vi "Construct Network Log Endpoint.vi"(8 "Max Number of Connections (-1)":i32=-1, 9 "Port":u16=7705, 10 "Net Address":u32, 11 "Logger to Write To":refnum<class "LoggerReference.lvclass">) -> (0 "error out":errorcluster, 3 "Network Sink Endpoint out":refnum<class "Network Sink Endpoint.lvclass">)   [LabVIEW 2017, in "Network Sink.lvlib" / "Network Sink Endpoint.lvclass"]
uses:
  <vilib>/gpm_packages/@cs/event-logger/Source/Network Sink/Network Sink Endpoint/Network Sink Endpoint.lvclass
  <vilib>/gpm_packages/@cs/event-logger/Source/Composed Log/LoggerReference/LoggerReference.lvclass
  <vilib>/gpm_packages/@cs/event-logger/Source/Network Sink/Network Sink Endpoint/Network Sink Endpoint.lvclass/Network Sink Endpoint.ctl
panel:
  # "The sink endpoint will stop itself with the logger shutdown - this output is only needed if you want to explicitly close the endpoint."
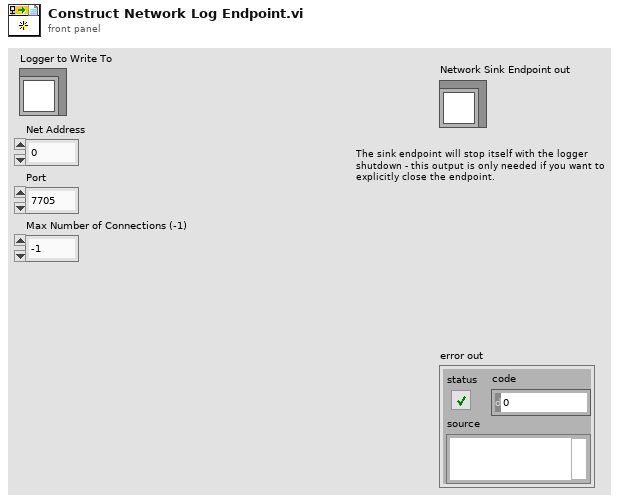
[diagram p1: front panel]
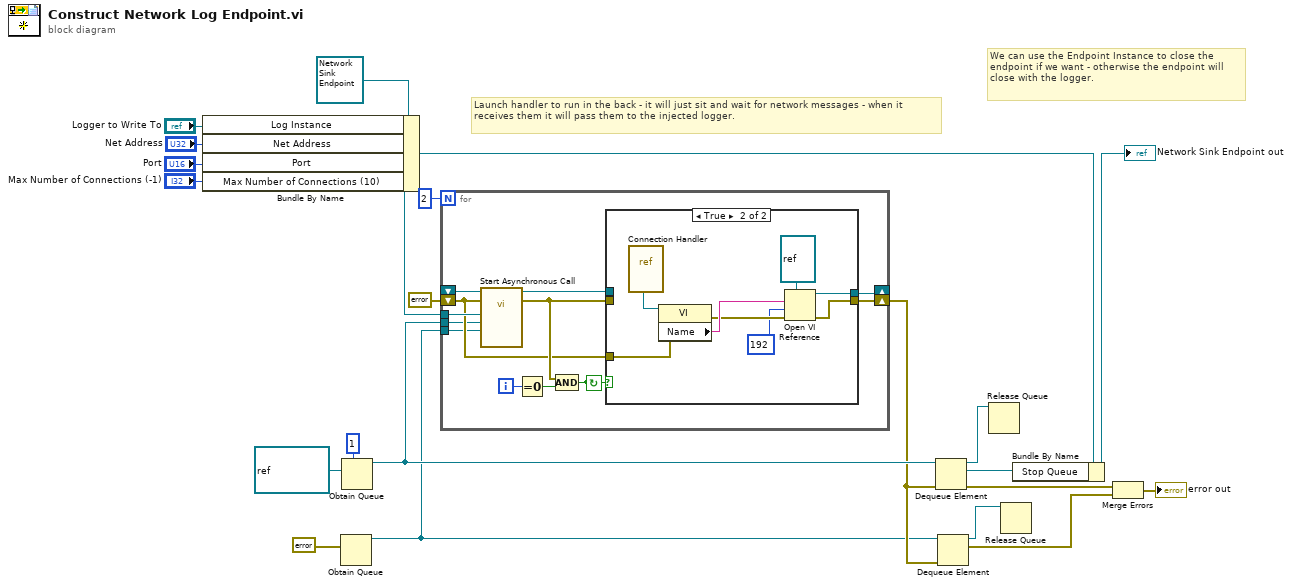
[diagram p0: block diagram]
diagram:
  # "We can use the Endpoint Instance to close the endpoint if we want - otherwise the endpoint will close with the logger."
  # "Launch handler to run in the back - it will just sit and wait for network messages - when it receives them it will pass them to the injected logger."
  n1 = Bundle By Name(cluster=refnum<class "Network Sink Endpoint.lvclass"> refnum ("Network Sink Endpoint in"), "Log Instance"="Logger to Write To", "Net Address"="Net Address", "Port"="Port", "Max Number of Connections (10)"="Max Number of Connections (-1)") -> (w16:refnum<class "Network Sink Endpoint.lvclass">)
  n2 = Obtain Queue(element data type=errorcluster {"status"=FALSE, "code"=0, "source"=""} ("error out")) -> (queue out=w5:refnum<queue>)  [unwired: 4 in, 2 out]
  n3 = Obtain Queue(max queue size (-1, unlimited)=1, element data type=refnum<queue> refnum ("Stop Queue")) -> (queue out=w14:refnum<queue>)  [unwired: 3 in, 2 out]
  n4 = for {
    N: 2 -> [_]
    tunnel: w16 -> [w26]
    shift-right: [w32] -> _
    shift-left: _ -> [w33]
    shift-right: [w27] -> w6
    shift-left: errorcluster {"status"=FALSE, "code"=0, "source"=""} ("error out") -> [w25]
    tunnel: w14 -> [w23]
    tunnel: w5 -> [w22]
    i -> [w29]
    stop <- w24 continue-if-true
    n5 = call-by-ref "Start Asynchronous Call"(reference=w33, error in=w25, "Error Return"=w22, "Return Queue"=w23, "Network Sink Endpoint in"=w26) -> (reference out=w31:refnum<vi>, error out=w28:errorcluster)  [unwired: 9 in]
    n6 = Equal To 0?(x=w29) -> (x = 0?=w30:bool)
    n7 = Compound Arithmetic op=AND(w28, w30) -> (w24:bool)
    n8 = case shown="True" w24 {
      tunnel: [w35 w40] -> w32
      tunnel: w31 -> [w35 _]
      tunnel: w28 -> [w34 _]
      tunnel: [w34 w38] -> w27
      tunnel: w25 -> [_ w37]
      frame False {
      }
      frame True {
        n9 = vi-ref <vilib>:"Connection Handler.vi"() -> (w43:refnum<vi>)
        n10 = property class="VI"(reference=w43, error in=w37) -> (error out=w39:errorcluster, "Name"=w42:string)  [unwired: 1 out]
        n11 = Open VI Reference(type specifier VI Refnum (for type only)=refnum<vi> refnum, vi path=w42, options=192 ("options: Multiple Clones,\n  Fire & Forget"), error in (no error)=w39) -> (vi reference=w40:refnum<vi>, error out=w38:errorcluster)  [unwired: 2 in]
      }
    }
  }
  n12 = Dequeue Element(queue=w14, error in (no error)=w6) -> (queue out=w8:refnum<queue>, element=w12:refnum<queue>, error out=w11:errorcluster)  [unwired: 1 in, 1 out]
  n13 = Dequeue Element(queue=w5, error in (no error)=w6) -> (queue out=w4:refnum<queue>, element=w2:errorcluster)  [unwired: 1 in, 2 out]
  n14 = Release Queue(queue=w8) -> ()  [unwired: 2 in, 3 out]
  n15 = Release Queue(queue=w4) -> ()  [unwired: 2 in, 3 out]
  n16 = Bundle By Name(cluster=w16, "Stop Queue"=w12) -> (→"Network Sink Endpoint out":refnum<class "Network Sink Endpoint.lvclass">)
  n17 = Merge Errors(w11, w2) -> (→"error out":errorcluster)
